vi "Get All Tags.vi"(7 "Filter (none)":string, 8 "error in (no error)":errorcluster) -> (0 "error out":errorcluster, 1 "Tag Refs":refnum<data-value>[](array[refnum]), 2 "Tag Names":string[](array[string]))   [LabVIEW 2020, in "Tag Engine.lvlib"]
doc: "Return a list of all Tag Names and references.\n\nOptionally specify a filter. Only matched Tag names will be returned. Standard \"Match Pattern\" syntax applies. Match is not case sensitive."
uses:
  Tag Engine.lvlib
  Tag/Tag.lvclass
  Tag/Tag.lvclass/Tag.ctl
  Core/Tag Core.lvclass
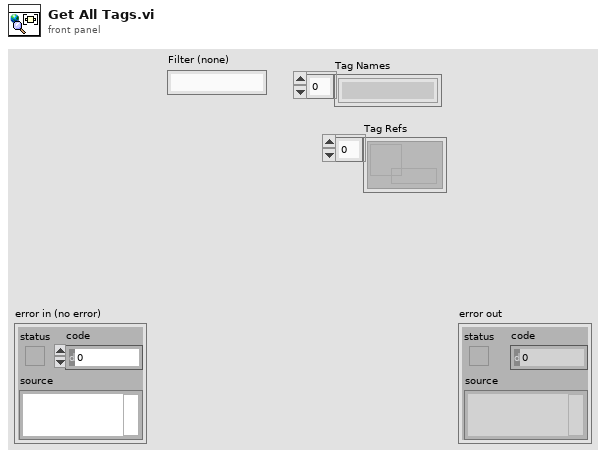
[diagram p1: front panel]
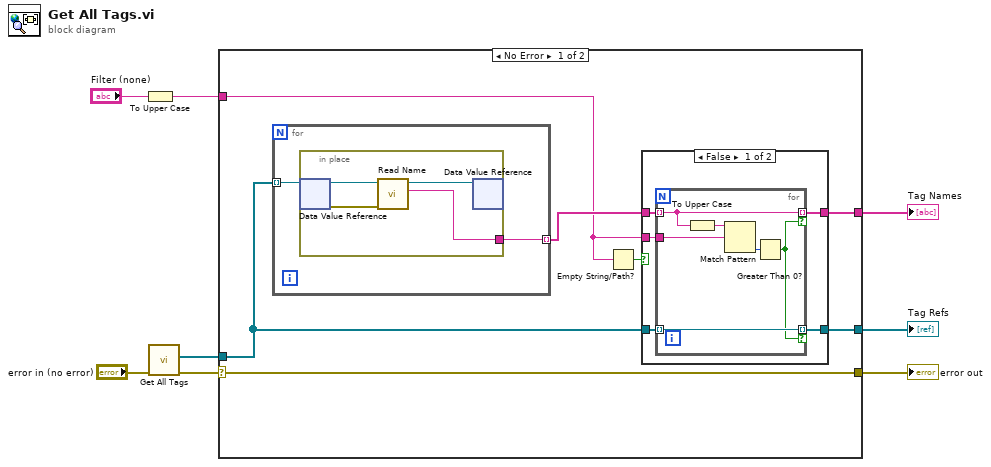
[diagram p0: block diagram]
diagram:
  n1 = To Upper Case(1:"Filter (none)") -> (0:w4:string)
  n2 = call "Get All Tags.vi"("error in (no error)"="error in (no error)") -> ("error out"=w2:errorcluster, "Tag Refs"=w1:refnum<data-value>[])  [unwired: 9 in]
  n3 = case shown="No Error" w2 {
    selector: w2 -> [w9 w35]
    tunnel: [w9 w35] -> w8
    tunnel: w1 -> [w10 _]
    tunnel: [w12 _] -> w6
    tunnel: [w11 _] -> w7
    tunnel: w4 -> [w13 _]
    frame No Error {
      n4 = for {
        tunnel: w10 -> [w30] mode=indexing
        tunnel: [w29] -> w14 mode=indexing
        n5 = in-place {
          in-place-border: [w32] -> w29
          n6 = in-place-dvr #1(w30) -> (w34:refnum<class "Tag.lvclass">, w31:errorcluster)
          n7 = call "Read Name.vi"("error in (no error)"=w31, "Tag in"=w34) -> ("Name"=w32:string, "Tag out"=w33:refnum<class "Tag.lvclass">)  [unwired: 7 in, 1 out]
          n8 = in-place-dvr #1(w33) -> ()  [unwired: 2 out]
        }
      }
      n9 = Empty String/Path?(string/path=w13) -> (empty?=w15:bool)
      n10 = case shown="False" w15 {
        tunnel: w14 -> [w20 w28]
        tunnel: [w19 w28] -> w12
        tunnel: w13 -> [w18 _]
        tunnel: w10 -> [w17 w27]
        tunnel: [w16 w27] -> w11
        frame False {
          n11 = for {
            tunnel: w18 -> [w26]
            tunnel: w20 -> [w24] mode=indexing
            tunnel: [w24] -> w19 mode=indexing if=w21
            tunnel: w17 -> [w22] mode=indexing
            tunnel: [w22] -> w16 mode=indexing if=w21
            n12 = To Upper Case(1:w24) -> (0:w23:string)
            n13 = Match Pattern(string=w23, regular expression=w26) -> (offset past match=w25:i32)  [unwired: 1 in, 3 out]
            n14 = Greater Than 0?(x=w25) -> (x > 0?=w21:bool)
          }
        }
        frame True {
        }
      }
    }
    frame Error {
    }
  }
  "error out" <- w8
  "Tag Refs" <- w7
  "Tag Names" <- w6
